vi "obstacle drawing.vi"(6 "color(black)":u32(colorbox), 9 "picture":picture, 10 "Col input":dbl, 11 "Row input":dbl) -> (2 "new picture":picture)   [LabVIEW 2016]
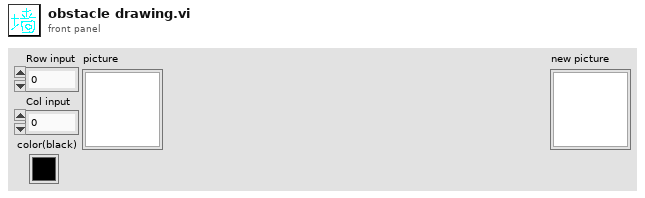
[diagram p1: front panel]
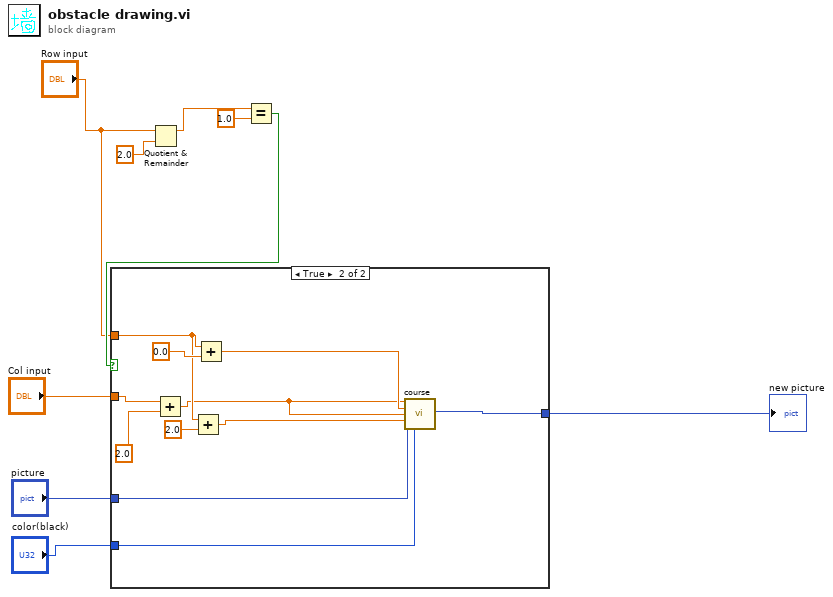
[diagram p0: block diagram]
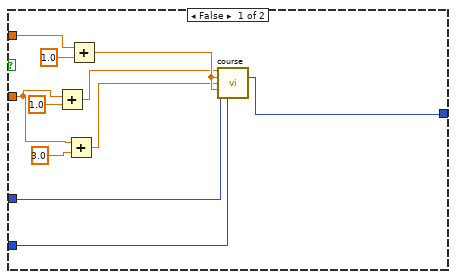
[diagram p2: hidden frame]
diagram:
  n1 = Quotient & Remainder(x="Row input", y=2.0) -> (x-y*floor(x/y)=w8:dbl)  [unwired: 1 out]
  n2 = Equal?(x=w8, y=1.0) -> (x = y?=w6:bool)
  n3 = case shown="True" w6 {
    tunnel: "Row input" -> [w17 w29]
    tunnel: "Col input" -> [w14 w25]
    tunnel: "picture" -> [w19 w28]
    tunnel: [w20 w27] -> w2
    tunnel: "color(black)" -> [w10 w21]
    frame False {
      n4 = Add(x=w14, y=1.0) -> (x+y=w12:dbl)
      n5 = Add(x=w14, y=3.0) -> (x+y=w11:dbl)
      n6 = Add(x=w17, y=1.0) -> (x+y=w13:dbl)
      n7 = call "course.vi"("x1"=w12, "y 1"=w13, "x2"=w11, "y 2"=w13, "picture"=w19, "color(black)"=w10) -> ("new picture"=w20:picture)  [unwired: 9 in]
    }
    frame True {
      n8 = Add(x=w25, y=2.0) -> (x+y=w22:dbl)
      n9 = Add(x=w29, y=2.0) -> (x+y=w23:dbl)
      n10 = Add(x=w29, y=0.0) -> (x+y=w24:dbl)
      n11 = call "course.vi"("x1"=w22, "y 1"=w24, "x2"=w22, "y 2"=w23, "picture"=w28, "color(black)"=w21) -> ("new picture"=w27:picture)  [unwired: 9 in]
    }
  }
  "new picture" <- w2
